vi "FlowThroughNMR.vi"() -> ()   [LabVIEW 2020]
uses:
  <instrlib>/niFgen/niFgen.llb/niFgen Output Mode.ctl
  <vilib>/Utility/file.llb/Write Delimited Spreadsheet (DBL).vi
panel:
  out "Scan Number 2":i32=8
  in  "Data points per iteration":dbl
  in  "File Folder for Data":string
  out "size(s)":i32
  out "Numeric":dbl
  in  "Write Output to File?":bool=TRUE
  out "Averaged T2 Decay":waveform(dbl)(graph)={"t0"=timestamp(0 s since 1904-01-01), "dt"=0.0012610340479192938, "Y"=array[3965 elements]} caption="Waveform Graph"
  in  "Number of Scans":i32=8
  out "Signal Intensity (Integral)":dbl=0.6544283602926818 format="%0.4f"
  out "Scan Number":i32=8
  out "Final Larmor Frequency":dbl format="%#_10g"
  in  "Pulse Train File":path=path "C:/Users/localuser/OneDrive - University of South Carolina/NMR Research/MATLAB/6 us 90 Degree - 1.25ms Tau - 3965 Pulses.txt"
  in  "Initial Larmor Frequency":dbl=27410000.0 caption="Frequency" format="%.3p"
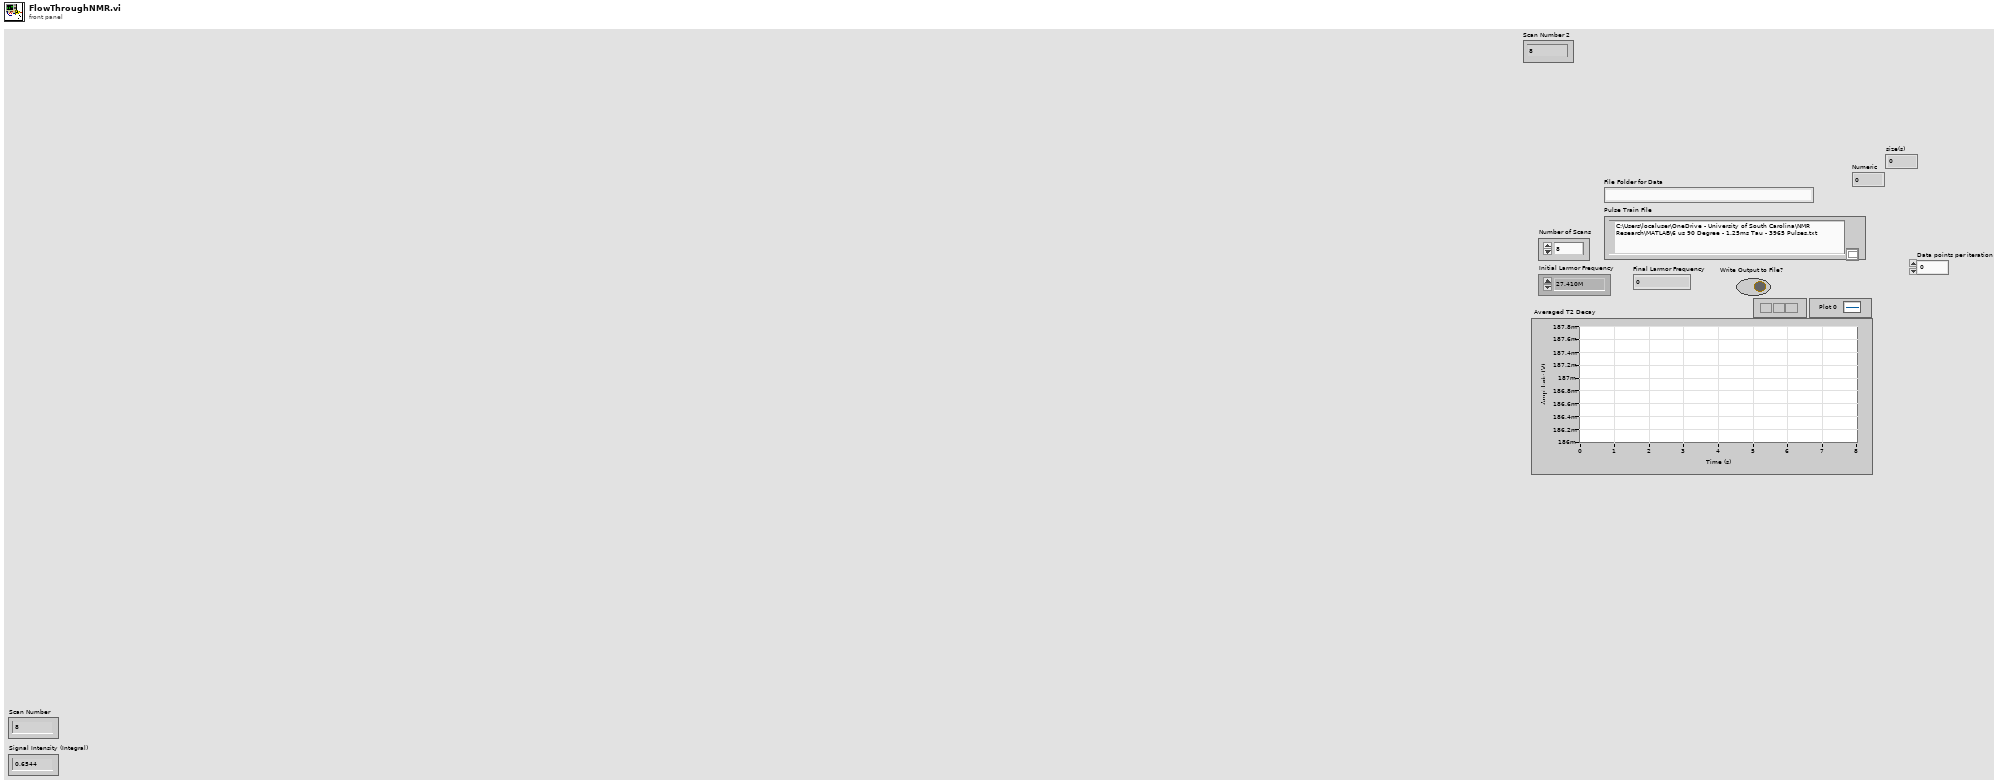
[diagram p1: front panel]
types:
  T1 = typedef "niFgen Output Mode.ctl" = u32
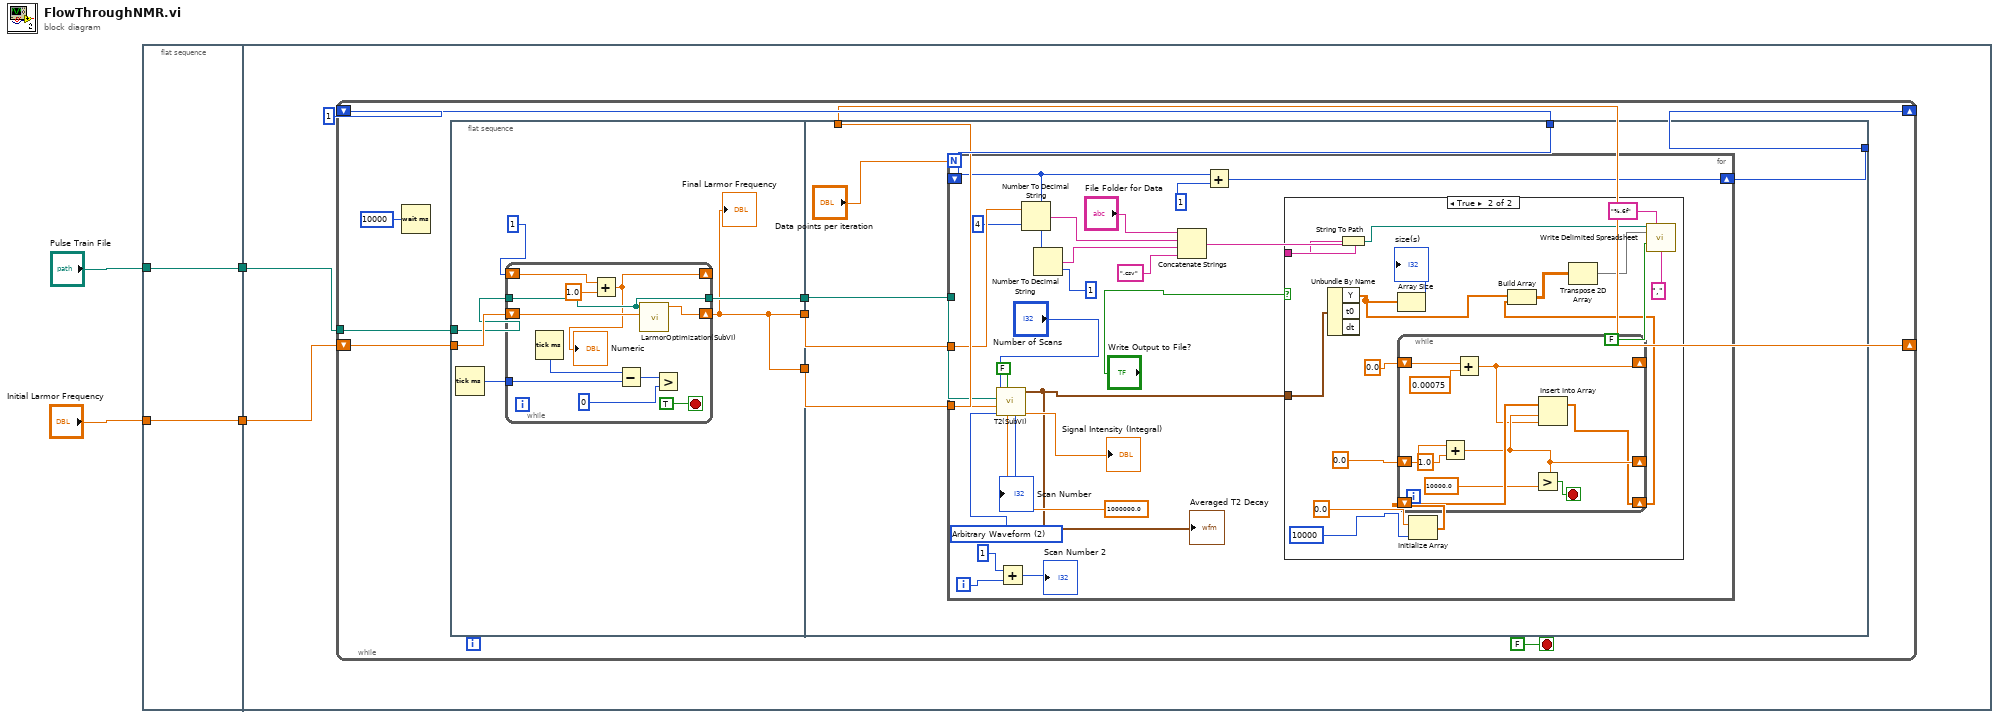
[diagram p0: block diagram]
diagram:
  n1 = flat-sequence {
    tunnel: "Pulse Train File" -> [w5]
    tunnel: "Initial Larmor Frequency" -> [w6]
    tunnel: [w6] -> w2
    tunnel: [w5] -> w1
    tunnel: w2 -> [w9]
    tunnel: w1 -> [w8]
    frame #0 {
    }
    frame #1 {
      n2 = while {
        tunnel: w8 -> [w18]
        shift-right: [w15] -> _
        shift-left: 1 -> [w16]
        shift-right: [w12] -> _
        shift-left: w9 -> [w19]
        stop <- FALSE stop-if-true
        n3 = Wait (ms)(milliseconds to wait=u32 10000) -> ()  [unwired: 1 out]
        n4 = flat-sequence {
          tunnel: w18 -> [w24]
          tunnel: w19 -> [w25]
          tunnel: [w20] -> w14
          tunnel: [w22] -> w13
          tunnel: [w20] -> w10
          tunnel: w16 -> [w42]
          tunnel: [w41] -> w15
          tunnel: w14 -> [w39]
          tunnel: w13 -> [w40]
          tunnel: [w39] -> w12
          tunnel: w10 -> [w38]
          frame #0 {
            n5 = Tick Count (ms)() -> (millisecond timer value=w23:u32)
            n6 = while {
              shift-right: [w36] -> w20
              shift-left: w25 -> [w35]
              tunnel: w24 -> [w30]
              tunnel: w23 -> [w32]
              tunnel: [w30] -> w22
              shift-right: [w27] -> _
              shift-left: 1 -> [w28]
              stop <- TRUE stop-if-true
              n7 = Tick Count (ms)() -> (millisecond timer value=w33:u32)
              n8 = Add(x=w28, y=1.0) -> (x+y=w27:dbl)
              "Numeric" <- w27
              n9 = Subtract(x=w33, y=w32) -> (x-y=w31:u32)
              n10 = call "LarmorOptimization(SubVI).vi"("Initial Larmor Frequency"=w35, "Pulse Train File in"=w30) -> ("Larmor Frequency 3"=w36:dbl)  [unwired: 9 in]
              n11 = Greater?(x=w31, y=u32 0) -> ()  [unwired: 1 out]
            }
            "Final Larmor Frequency" <- w20
          }
          frame #1 {
            n12 = for {
              N: "Data points per iteration" -> [_]
              tunnel: w40 -> [w55]
              tunnel: w39 -> [w52]
              tunnel: w38 -> [w51]
              shift-right: [w56] -> w41
              shift-left: w42 -> [w58]
              i -> [w45]
              w63 = T1 2 items=["Standard Function", "Frequency List", "Arbitrary Waveform", "Arbitrary Sequence", "Script"] ("output mode")
              n13 = call "T2(SubVI).vi"("Sample Rate"=1000000.0, "Write Output to File?"=FALSE, "output mode"=w63, "Larmor Frequency"=w52, "Pulse Train File"=w55, "Number of Scans"="Number of Scans") -> ("Signal Intensity (Integral)"=→"Signal Intensity (Integral)":dbl, "Averaged T2 Decay"=w47:waveform(dbl), "Scan Number"=→"Scan Number":i32)  [unwired: 3 out]
              "Averaged T2 Decay" <- w47
              n14 = Add(x=1, y=w45) -> (x+y=→"Scan Number 2":i32)
              n15 = Number To Decimal String(number=w51, width (-)=i16 4) -> (decimal integer string=w48:string)
              n16 = Number To Decimal String(number=w58, width (-)=i16 1) -> (decimal integer string=w53:string)
              n17 = Concatenate Strings("File Folder for Data", w48, w53, ".csv" ("string")) -> (w54:string)
              n18 = Add(x=w58, y=1) -> (x+y=w56:i32)
              n19 = case shown="True" "Write Output to File?" {
                tunnel: w54 -> [_ w82]
                tunnel: w47 -> [_ w78]
                frame False {
                }
                frame True {
                  n20 = Unbundle By Name(w78) -> ("Y"=w71:dbl[])  [unwired: 2 out]
                  n21 = String To Path(string=w82) -> (path=w81:path)
                  n22 = Array Size(array=w71) -> (size(s)=→"size(s)":i32)
                  n23 = Initialize Array(0.0 ("element"), 10000 ("dimension size")) -> (w76:dbl[])
                  n24 = while {
                    shift-right: [w83] -> _
                    shift-left: 0.0 -> [w90]
                    shift-right: [w85] -> _
                    shift-left: 0.0 -> [w86]
                    shift-right: [w84] -> w70
                    shift-left: w76 -> [w89]
                    stop <- w88 stop-if-true
                    n25 = Add(x=w86, y=1.0) -> (x+y=w85:dbl)
                    n26 = Add(x=w90, y=0.00075) -> (x+y=w83:dbl)
                    n27 = Greater?(x=w85, y=10000.0) -> (0:w88:bool)
                    n28 = Insert Into Array(array=w89, index=w85, new element=w83) -> (w84:dbl[])
                  }
                  n29 = Build Array(w71, w70) -> (w69:dbl[][])
                  n30 = Transpose 2D Array(2D array=w69) -> (transposed array=w68:dbl[][])
                  n31 = call-poly <vilib>:"Write Delimited Spreadsheet.vi"("file path (dialog if empty)"=w81, "format (%.3f)"="%.6f", "2D data"=w68, "append to file? (new file:F)"=FALSE, "delimiter (\\t)"="," ("delimiter (\\t)")) -> ()  [unwired: 9 in, 2 out]
                }
              }
            }
          }
        }
      }
    }
  }
